vi "conv2mat.vi"(0 "Ref Num":refnum<file>, 1 "Array name":string, 5 "pos mode (rel. to end: 1)":i16(ring)=1 items=["relative to beginning of file", "relative to end of file", "relative to current mark"], 7 "pos offset (bytes:0)":i32, 9 "Data Type (0:double)":T1(ring), 11 "error in (no error)":errorcluster, 12 "1D-array":cdb[](array[numeric]) format="%.2f", 13 "2D-array":cdb[][](array[numeric]) format="%.2f", 14 "String":string) -> (4 "Dup Ref Num":refnum<file>, 8 "mark after write (bytes)":i32, 15 "error out":errorcluster)   [LabVIEW 2015]
doc: "CONV2MAT.VI exports an array to Matlab format (.MAT file) at the specified location. The default location is at the end of file. The user will have to open the output file before and close it afterwards. The VI does incoming and internal error checking and does not write if an incoming error occurs.\n\nConnect the following terminals:\n- Ref number\n- array name; this name will also apear when the resulting file is read\n into Matlab.\n- Data type; this specifies the output data type. This can come in\n handy if you want to reduce the output file size.\n- either 1D-array, 2D-array or String. If you want to write a string,\n do not connect Data Type (caracters will be converted to floating\n point numbers representing their ASCII-value).\n\nPos mode and Pos offset default to write any data at the end of the file.\n\nAlbert K. Wijnja\nUniversity of Technology Eindhoven\nE-mail: albert@wfw.wtb.tue.nl\n\nSeptember 1994"
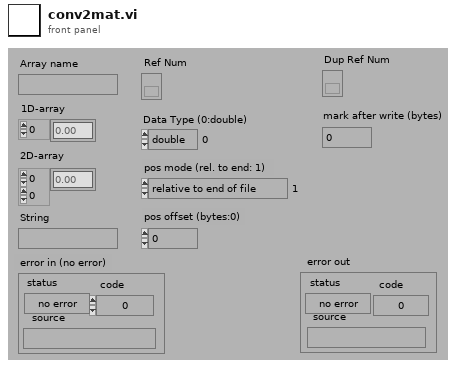
[diagram p1: front panel]
types:
  T1 = enum16{"double", "single", "int 32", "int 16", "u-int 16", "u-int 8"}
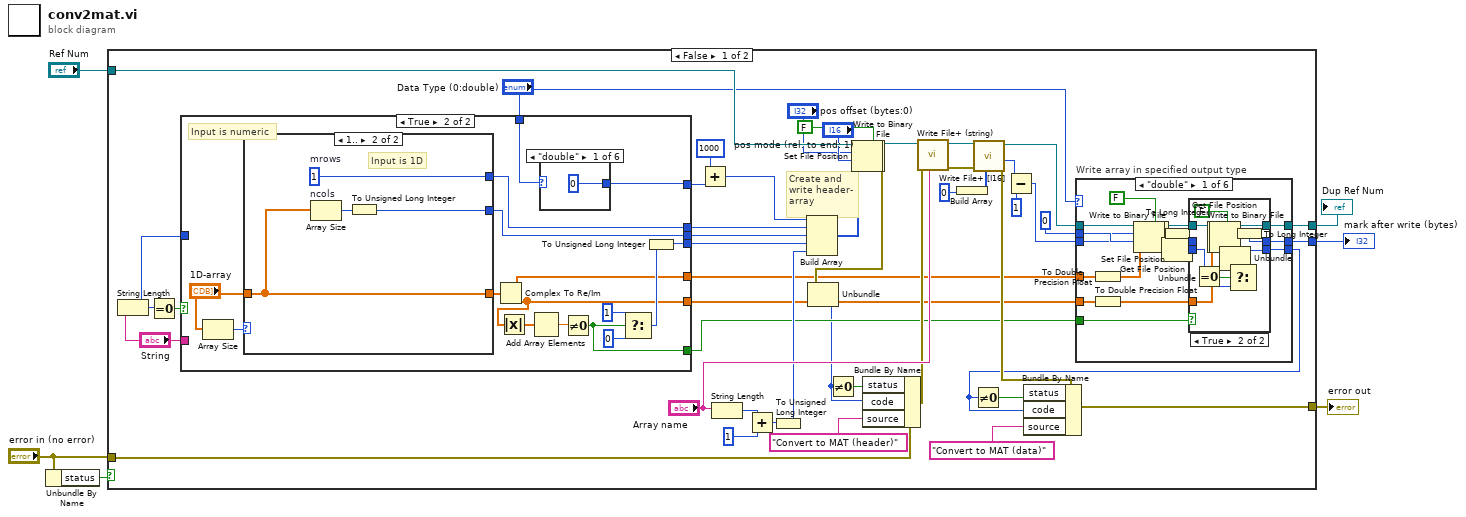
[diagram p0: block diagram]
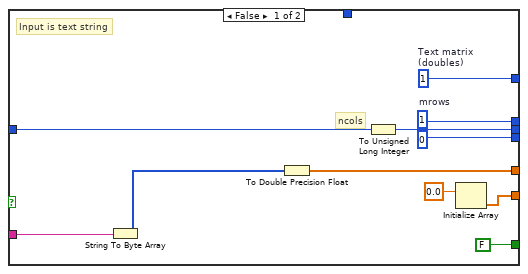
[diagram p2: hidden frame]
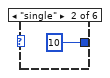
[diagram p3: hidden frame]
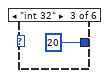
[diagram p4: hidden frame]
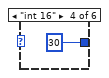
[diagram p5: hidden frame]
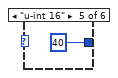
[diagram p6: hidden frame]
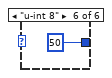
[diagram p7: hidden frame]
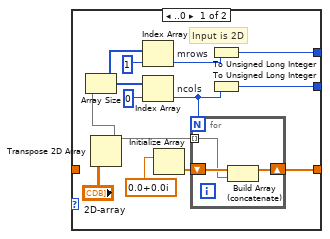
[diagram p8: hidden frame]
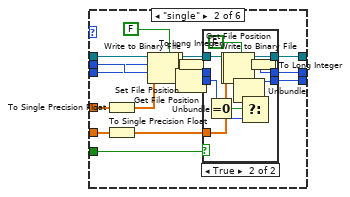
[diagram p10: hidden frame]
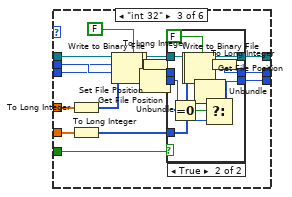
[diagram p12: hidden frame]
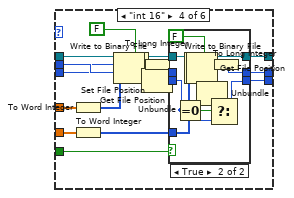
[diagram p14: hidden frame]
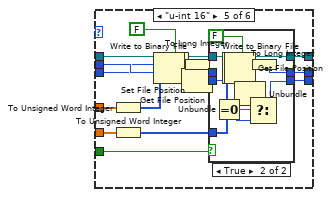
[diagram p16: hidden frame]
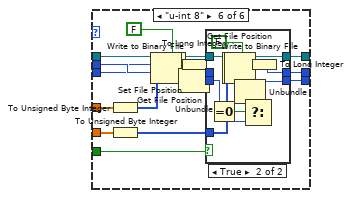
[diagram p18: hidden frame]
diagram:
  n1 = Unbundle By Name("error in (no error)") -> ("status"=w6:bool)
  n2 = case shown="False" w6 {
    tunnel: [w30 w331] -> w4
    tunnel: [w27 w330] -> w2
    tunnel: "Ref Num" -> [w39 w330]
    tunnel: "error in (no error)" -> [w52 w331]
    tunnel: [w26 -1] -> w1
    frame False {
      # "Create and\nwrite header-\narray"
      n3 = String Length(string="String") -> (length=w21:i32)
      n4 = Equal To 0?(x=w21) -> (x = 0?=w23:bool)
      n5 = case shown="True" w23 {
        tunnel: [w58 w74] -> w16
        tunnel: [w60 w67] -> w15
        tunnel: "String" -> [w61 _]
        tunnel: [w56 w73] -> w20
        tunnel: [w64 w72] -> w19
        tunnel: [FALSE w71] -> w18
        tunnel: [u32 0 w70] -> w17
        tunnel: w21 -> [w65 _]
        tunnel: [w57 w69] -> w13
        tunnel: "Data Type (0:double)" -> [_ w68]
        frame False {
          w57 = u32 1  # Text matrix (doubles)
          w56 = u32 1  # mrows
          # "Input is text string"
          # "ncols"
          n6 = String To Byte Array(string=w61) -> (unsigned byte array=w59:u8[])
          n7 = To Double Precision Float(number=w59) -> (double precision float=w58:dbl[])
          n8 = To Unsigned Long Integer(number=w65) -> (unsigned 32bit integer=w64:u32)
          n9 = Initialize Array(0.0) -> (w60:dbl[])  [unwired: 1 in]
        }
        frame True {
          # "Input is numeric"
          n10 = Array Size(array="1D-array") -> (size(s)=w75:i32)
          n11 = case shown="1.." w75 {
            tunnel: "1D-array" -> [_ w106]
            tunnel: [w92 w106] -> w79
            tunnel: [w91 w103] -> w73
            tunnel: [w90 w104] -> w72
            frame ..0 {
              # "Input is 2D"
              n12 = Transpose 2D Array(2D array="2D-array") -> (transposed array=w99:cdb[][])
              n13 = Array Size(array=w99) -> (size(s)=w98:i32[])
              n14 = Index Array "mrows"(array=w98, index=1) -> (element=w94:i32)
              n15 = Index Array "ncols"(array=w98, index=0) -> (element=w95:i32)
              n16 = Initialize Array(cdb 0.0+0.0i) -> (w93:cdb[])  [unwired: 1 in]
              n17 = for {
                N: w95 -> [_]
                tunnel: w99 -> [w100] mode=indexing
                shift-right: [w101] -> w92
                shift-left: w93 -> [w102]
                n18 = Build Array (concatenate)(w102, w100) -> (w101:cdb[])
              }
              n19 = To Unsigned Long Integer(number=w94) -> (unsigned 32bit integer=w91:u32)
              n20 = To Unsigned Long Integer(number=w95) -> (unsigned 32bit integer=w90:u32)
            }
            frame 1.. {
              w103 = u32 1  # mrows
              # "Input is 1D"
              n21 = Array Size "ncols"(array=w106) -> (size(s)=w105:i32)
              n22 = To Unsigned Long Integer(number=w105) -> (unsigned 32bit integer=w104:u32)
            }
          }
          n23 = Complex To Re/Im(x + iy=w79) -> (x=w74:dbl[], y=w67:dbl[])
          n24 = Absolute Value(x=w67) -> (abs(x)=w66:dbl[])
          n25 = Add Array Elements(numeric array=w66) -> (sum=w81:dbl)
          n26 = case shown="\"double\"" w68 {
            tunnel: [u32 0 u32 10 u32 20 u32 30 u32 40 u32 50] -> w69
            frame "double" {
            }
            frame "single" {
            }
            frame "int 32" {
            }
            frame "int 16" {
            }
            frame "u-int 16" {
            }
            frame "u-int 8" {
            }
          }
          n27 = Not Equal To 0?(x=w81) -> (x != 0?=w71:bool)
          n28 = Select(t=1, s=w71, f=0) -> (s? t:f=w78:i32)
          n29 = To Unsigned Long Integer(number=w78) -> (unsigned 32bit integer=w70:u32)
        }
      }
      n30 = Add(x=u32 1000, y=w13) -> (x+y=w12:u32)
      n31 = String Length(string="Array name") -> (length=w50:i32)
      n32 = Add(x=w50, y=1) -> (x+y=w48:i32)
      n33 = To Unsigned Long Integer(number=w48) -> (unsigned 32bit integer=w47:u32)
      n34 = Build Array(w12, w20, w19, w17, w47) -> (w36:u32[])
      n35 = Set File Position(offset (in bytes) (0)="pos offset (bytes:0)", refnum=w39, from (0:start)="pos mode (rel. to end: 1)") -> (refnum out=w9:refnum<file>, error out=w8:errorcluster)  [unwired: 1 in]
      n36 = Write to Binary File(file (use dialog)=w9, data=w36, error in=w8, 5:FALSE ("prepend array or string size? (T)")) -> (refnum out=w46:refnum<file>, error out=w35:errorcluster)  [unwired: 2 in, 1 out]
      n37 = Unbundle(w35) -> ("code"=w10:i32)  [unwired: 2 out]
      n38 = Not Equal To 0?(x=w10) -> (x != 0?=w54:bool)
      n39 = Bundle By Name(cluster=w52, "status"=w54, "code"=w10, "source"="Convert to MAT (header)") -> (w34:errorcluster)
      n40 = call <vilib>:"Write File+ (string).vi"("string"="Array name", "error in (no error)"=w34, "refnum"=w46) -> ("error out"=w41:errorcluster, "dup refnum"=w40:refnum<file>)  [unwired: 4 in, 1 out]
      n41 = Build Array(u8 0) -> (w43:u8[])
      n42 = call <vilib>:"Write File+ [I16].vi"("1D array"=w43, "error in (no error)"=w41, "refnum"=w40) -> ("error out"=w31:errorcluster, "mark after write (bytes)"=w45:i32, "dup refnum"=w28:refnum<file>)  [unwired: 6 in]
      n43 = Subtract(x=w45, y=1) -> (x-y=w25:i32)
      n44 = case "Write array in specified output type" shown="\"double\"" "Data Type (0:double)" {
        tunnel: w16 -> [w115 w152 w189 w226 w263 w300]
        tunnel: i16 0 -> [w124 w161 w198 w235 w272 w309]
        tunnel: w28 -> [w125 w162 w199 w236 w273 w310]
        tunnel: [w127 w164 w201 w238 w275 w312] -> w27
        tunnel: [w126 w163 w200 w237 w274 w311] -> w26
        tunnel: w25 -> [w123 w160 w197 w234 w271 w308]
        tunnel: w15 -> [w114 w151 w188 w225 w262 w299]
        tunnel: w18 -> [w116 w153 w190 w227 w264 w301]
        tunnel: [w117 w154 w191 w228 w265 w302] -> w24
        frame "double" {
          n45 = To Double Precision Float(number=w115) -> (double precision float=w122:dbl[])
          n46 = To Double Precision Float(number=w114) -> (double precision float=w119:dbl[])
          n47 = Set File Position(offset (in bytes) (0)=w123, refnum=w125, from (0:start)=w124) -> (refnum out=w112:refnum<file>, error out=w111:errorcluster)  [unwired: 1 in]
          n48 = Write to Binary File(file (use dialog)=w112, data=w122, error in=w111, 5:FALSE ("prepend array or string size? (T)")) -> (refnum out=w110:refnum<file>, error out=w109:errorcluster)  [unwired: 2 in, 1 out]
          n49 = Get File Position(4:w109, 7:w110) -> (0:w118:errorcluster, 2:w108:i64, 3:w120:refnum<file>)
          n50 = To Long Integer(number=w108) -> (32bit integer=w121:i32)
          n51 = Unbundle(w118) -> ("code"=w113:i32)  [unwired: 2 out]
          n52 = case shown="True" w116 {
            tunnel: [w130 w141] -> w127
            tunnel: w120 -> [w130 w143]
            tunnel: [w129 w140] -> w126
            tunnel: w121 -> [w129 _]
            tunnel: w119 -> [_ w142]
            tunnel: [w128 w138] -> w117
            tunnel: w113 -> [w128 w136]
            frame False {
            }
            frame True {
              n53 = Equal To 0?(x=w136) -> (x = 0?=w139:bool)
              n54 = Write to Binary File(file (use dialog)=w143, data=w142, 5:FALSE ("prepend array or string size? (T)")) -> (refnum out=w134:refnum<file>, error out=w133:errorcluster)  [unwired: 3 in, 1 out]
              n55 = Get File Position(4:w133, 7:w134) -> (0:w137:errorcluster, 2:w132:i64, 3:w141:refnum<file>)
              n56 = Unbundle(w137) -> ("code"=w135:i32)  [unwired: 2 out]
              n57 = Select(t=w135, s=w139, f=w136) -> (s? t:f=w138:i32)
              n58 = To Long Integer(number=w132) -> (32bit integer=w140:i32)
            }
          }
        }
        frame "single" {
          n59 = To Single Precision Float(number=w152) -> (single precision float=w159:sgl[])
          n60 = To Single Precision Float(number=w151) -> (single precision float=w156:sgl[])
          n61 = Set File Position(offset (in bytes) (0)=w160, refnum=w162, from (0:start)=w161) -> (refnum out=w149:refnum<file>, error out=w148:errorcluster)  [unwired: 1 in]
          n62 = Write to Binary File(file (use dialog)=w149, data=w159, error in=w148, 5:FALSE ("prepend array or string size? (T)")) -> (refnum out=w147:refnum<file>, error out=w146:errorcluster)  [unwired: 2 in, 1 out]
          n63 = Get File Position(4:w146, 7:w147) -> (0:w155:errorcluster, 2:w145:i64, 3:w157:refnum<file>)
          n64 = To Long Integer(number=w145) -> (32bit integer=w158:i32)
          n65 = Unbundle(w155) -> ("code"=w150:i32)  [unwired: 2 out]
          n66 = case shown="True" w153 {
            tunnel: [w167 w178] -> w164
            tunnel: w157 -> [w167 w180]
            tunnel: [w166 w177] -> w163
            tunnel: w158 -> [w166 _]
            tunnel: w156 -> [_ w179]
            tunnel: [w165 w173] -> w154
            tunnel: w150 -> [w165 w175]
            frame False {
            }
            frame True {
              n67 = Equal To 0?(x=w175) -> (x = 0?=w176:bool)
              n68 = Write to Binary File(file (use dialog)=w180, data=w179, 5:FALSE ("prepend array or string size? (T)")) -> (refnum out=w171:refnum<file>, error out=w170:errorcluster)  [unwired: 3 in, 1 out]
              n69 = Get File Position(4:w170, 7:w171) -> (0:w174:errorcluster, 2:w169:i64, 3:w178:refnum<file>)
              n70 = Unbundle(w174) -> ("code"=w172:i32)  [unwired: 2 out]
              n71 = Select(t=w172, s=w176, f=w175) -> (s? t:f=w173:i32)
              n72 = To Long Integer(number=w169) -> (32bit integer=w177:i32)
            }
          }
        }
        frame "int 32" {
          n73 = To Long Integer(number=w189) -> (32bit integer=w196:i32[])
          n74 = To Long Integer(number=w188) -> (32bit integer=w193:i32[])
          n75 = Set File Position(offset (in bytes) (0)=w197, refnum=w199, from (0:start)=w198) -> (refnum out=w186:refnum<file>, error out=w185:errorcluster)  [unwired: 1 in]
          n76 = Write to Binary File(file (use dialog)=w186, data=w196, error in=w185, 5:FALSE ("prepend array or string size? (T)")) -> (refnum out=w184:refnum<file>, error out=w183:errorcluster)  [unwired: 2 in, 1 out]
          n77 = Get File Position(4:w183, 7:w184) -> (0:w192:errorcluster, 2:w182:i64, 3:w194:refnum<file>)
          n78 = To Long Integer(number=w182) -> (32bit integer=w195:i32)
          n79 = Unbundle(w192) -> ("code"=w187:i32)  [unwired: 2 out]
          n80 = case shown="True" w190 {
            tunnel: [w204 w215] -> w201
            tunnel: w194 -> [w204 w217]
            tunnel: [w203 w214] -> w200
            tunnel: w195 -> [w203 _]
            tunnel: w193 -> [_ w216]
            tunnel: [w202 w210] -> w191
            tunnel: w187 -> [w202 w212]
            frame False {
            }
            frame True {
              n81 = Equal To 0?(x=w212) -> (x = 0?=w213:bool)
              n82 = Write to Binary File(file (use dialog)=w217, data=w216, 5:FALSE ("prepend array or string size? (T)")) -> (refnum out=w208:refnum<file>, error out=w207:errorcluster)  [unwired: 3 in, 1 out]
              n83 = Get File Position(4:w207, 7:w208) -> (0:w211:errorcluster, 2:w206:i64, 3:w215:refnum<file>)
              n84 = Unbundle(w211) -> ("code"=w209:i32)  [unwired: 2 out]
              n85 = Select(t=w209, s=w213, f=w212) -> (s? t:f=w210:i32)
              n86 = To Long Integer(number=w206) -> (32bit integer=w214:i32)
            }
          }
        }
        frame "int 16" {
          n87 = To Word Integer(number=w226) -> (16bit integer=w233:i16[])
          n88 = To Word Integer(number=w225) -> (16bit integer=w230:i16[])
          n89 = Set File Position(offset (in bytes) (0)=w234, refnum=w236, from (0:start)=w235) -> (refnum out=w223:refnum<file>, error out=w222:errorcluster)  [unwired: 1 in]
          n90 = Write to Binary File(file (use dialog)=w223, data=w233, error in=w222, 5:FALSE ("prepend array or string size? (T)")) -> (refnum out=w221:refnum<file>, error out=w220:errorcluster)  [unwired: 2 in, 1 out]
          n91 = Get File Position(4:w220, 7:w221) -> (0:w229:errorcluster, 2:w219:i64, 3:w231:refnum<file>)
          n92 = To Long Integer(number=w219) -> (32bit integer=w232:i32)
          n93 = Unbundle(w229) -> ("code"=w224:i32)  [unwired: 2 out]
          n94 = case shown="True" w227 {
            tunnel: [w241 w252] -> w238
            tunnel: w231 -> [w241 w254]
            tunnel: [w240 w251] -> w237
            tunnel: w232 -> [w240 _]
            tunnel: w230 -> [_ w253]
            tunnel: [w239 w247] -> w228
            tunnel: w224 -> [w239 w249]
            frame False {
            }
            frame True {
              n95 = Equal To 0?(x=w249) -> (x = 0?=w250:bool)
              n96 = Write to Binary File(file (use dialog)=w254, data=w253, 5:FALSE ("prepend array or string size? (T)")) -> (refnum out=w245:refnum<file>, error out=w244:errorcluster)  [unwired: 3 in, 1 out]
              n97 = Get File Position(4:w244, 7:w245) -> (0:w248:errorcluster, 2:w243:i64, 3:w252:refnum<file>)
              n98 = Unbundle(w248) -> ("code"=w246:i32)  [unwired: 2 out]
              n99 = Select(t=w246, s=w250, f=w249) -> (s? t:f=w247:i32)
              n100 = To Long Integer(number=w243) -> (32bit integer=w251:i32)
            }
          }
        }
        frame "u-int 16" {
          n101 = To Unsigned Word Integer(number=w263) -> (unsigned 16bit integer=w270:u16[])
          n102 = To Unsigned Word Integer(number=w262) -> (unsigned 16bit integer=w267:u16[])
          n103 = Set File Position(offset (in bytes) (0)=w271, refnum=w273, from (0:start)=w272) -> (refnum out=w260:refnum<file>, error out=w259:errorcluster)  [unwired: 1 in]
          n104 = Write to Binary File(file (use dialog)=w260, data=w270, error in=w259, 5:FALSE ("prepend array or string size? (T)")) -> (refnum out=w258:refnum<file>, error out=w257:errorcluster)  [unwired: 2 in, 1 out]
          n105 = Get File Position(4:w257, 7:w258) -> (0:w266:errorcluster, 2:w256:i64, 3:w268:refnum<file>)
          n106 = To Long Integer(number=w256) -> (32bit integer=w269:i32)
          n107 = Unbundle(w266) -> ("code"=w261:i32)  [unwired: 2 out]
          n108 = case shown="True" w264 {
            tunnel: [w278 w289] -> w275
            tunnel: w268 -> [w278 w291]
            tunnel: [w277 w288] -> w274
            tunnel: w269 -> [w277 _]
            tunnel: w267 -> [_ w290]
            tunnel: [w276 w284] -> w265
            tunnel: w261 -> [w276 w286]
            frame False {
            }
            frame True {
              n109 = Equal To 0?(x=w286) -> (x = 0?=w287:bool)
              n110 = Write to Binary File(file (use dialog)=w291, data=w290, 5:FALSE ("prepend array or string size? (T)")) -> (refnum out=w282:refnum<file>, error out=w281:errorcluster)  [unwired: 3 in, 1 out]
              n111 = Get File Position(4:w281, 7:w282) -> (0:w285:errorcluster, 2:w280:i64, 3:w289:refnum<file>)
              n112 = Unbundle(w285) -> ("code"=w283:i32)  [unwired: 2 out]
              n113 = Select(t=w283, s=w287, f=w286) -> (s? t:f=w284:i32)
              n114 = To Long Integer(number=w280) -> (32bit integer=w288:i32)
            }
          }
        }
        frame "u-int 8" {
          n115 = To Unsigned Byte Integer(number=w300) -> (unsigned 8bit integer=w307:u8[])
          n116 = To Unsigned Byte Integer(number=w299) -> (unsigned 8bit integer=w304:u8[])
          n117 = Set File Position(offset (in bytes) (0)=w308, refnum=w310, from (0:start)=w309) -> (refnum out=w297:refnum<file>, error out=w296:errorcluster)  [unwired: 1 in]
          n118 = Write to Binary File(file (use dialog)=w297, data=w307, error in=w296, 5:FALSE ("prepend array or string size? (T)")) -> (refnum out=w295:refnum<file>, error out=w294:errorcluster)  [unwired: 2 in, 1 out]
          n119 = Get File Position(4:w294, 7:w295) -> (0:w303:errorcluster, 2:w293:i64, 3:w305:refnum<file>)
          n120 = To Long Integer(number=w293) -> (32bit integer=w306:i32)
          n121 = Unbundle(w303) -> ("code"=w298:i32)  [unwired: 2 out]
          n122 = case shown="True" w301 {
            tunnel: [w315 w326] -> w312
            tunnel: w305 -> [w315 w328]
            tunnel: [w314 w325] -> w311
            tunnel: w306 -> [w314 _]
            tunnel: w304 -> [_ w327]
            tunnel: [w313 w322] -> w302
            tunnel: w298 -> [w313 w323]
            frame False {
            }
            frame True {
              n123 = Equal To 0?(x=w323) -> (x = 0?=w324:bool)
              n124 = Write to Binary File(file (use dialog)=w328, data=w327, 5:FALSE ("prepend array or string size? (T)")) -> (refnum out=w319:refnum<file>, error out=w318:errorcluster)  [unwired: 3 in, 1 out]
              n125 = Get File Position(4:w318, 7:w319) -> (0:w321:errorcluster, 2:w317:i64, 3:w326:refnum<file>)
              n126 = Unbundle(w321) -> ("code"=w320:i32)  [unwired: 2 out]
              n127 = Select(t=w320, s=w324, f=w323) -> (s? t:f=w322:i32)
              n128 = To Long Integer(number=w317) -> (32bit integer=w325:i32)
            }
          }
        }
      }
      n129 = Not Equal To 0?(x=w24) -> (x != 0?=w32:bool)
      n130 = Bundle By Name(cluster=w31, "status"=w32, "code"=w24, "source"="Convert to MAT (data)") -> (w30:errorcluster)
    }
    frame True {
    }
  }
  "Dup Ref Num" <- w2
  "error out" <- w4
  "mark after write (bytes)" <- w1
